vi "counter 1 with semaphore.vi"() -> ()   [LabVIEW 2009]
panel:
  out "Compte 1":i32
  out "total cumulatif":i32
  in  "stop":bool
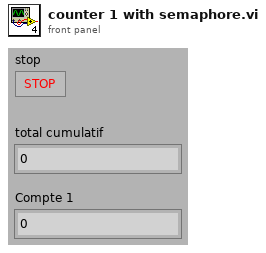
[diagram p1: front panel]
types:
  T1 = typedef "Semaphore RefNum" = refnum<k1>
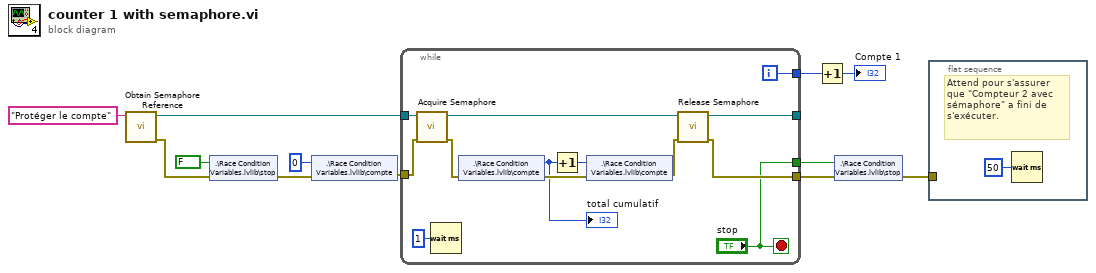
[diagram p0: block diagram]
diagram:
  n1 = call <vilib>:"Obtain Semaphore Reference.vi"("name (unnamed)"="Protéger le compte") -> ("error out"=w4:errorcluster, "semaphore"=w7:T1)  [unwired: 4 in, 1 out]
  n2 = shared-variable ".\\Race Condition Variables.lvlib\\stop"(FALSE ("stop"), error in=w4) -> (error out=w3:errorcluster)
  n3 = shared-variable ".\\Race Condition Variables.lvlib\\compte"(0 ("counter"), error in=w3) -> (error out=w12:errorcluster)
  n4 = while "Boucle While" {
    tunnel: [w24] -> w11
    tunnel: w12 -> [w19]
    tunnel: w7 -> [w20]
    tunnel: [w15] -> _
    tunnel: [w14] -> w6
    tunnel: ["stop"] -> w5
    i -> [w24]
    stop <- "stop" stop-if-true
    n5 = call <vilib>:"Acquire Semaphore.vi"("error in (no error)"=w19, "semaphore"=w20) -> ("error out"=w18:errorcluster, "semaphore out"=w16:T1)  [unwired: 3 in, 1 out]
    n6 = Wait (ms) ("Attendre (ms)")(milliseconds to wait=u32 1) -> ()  [unwired: 1 out]
    n7 = shared-variable ".\\Race Condition Variables.lvlib\\compte"(error in=w18) -> (w21:i32, error out=w25:errorcluster)
    "total cumulatif" <- w21
    n8 = Increment ("Incrémenter")(x=w21) -> (x+1=w22:i32)
    n9 = shared-variable ".\\Race Condition Variables.lvlib\\compte"(w22, error in=w25) -> (error out=w17:errorcluster)
    n10 = call <vilib>:"Release Semaphore.vi"("error in (no error)"=w17, "semaphore"=w16) -> ("error out"=w14:errorcluster, "semaphore out"=w15:T1)  [unwired: 4 in]
  }
  n11 = Increment ("Incrémenter")(x=w11) -> (x+1=→"Compte 1":i32)
  n12 = shared-variable ".\\Race Condition Variables.lvlib\\stop"(w5, error in=w6) -> (error out=w1:errorcluster)
  n13 = flat-sequence {
    tunnel: w1 -> [_]
    frame #0 {
      # "Attend pour s'assurer que \"Compteur 2 avec sémaphore\" a fini de s'exécuter."
      n14 = Wait (ms)(milliseconds to wait=u32 50) -> ()  [unwired: 1 out]
    }
  }
